vi "Destroy.vi"(8 "error in (no error)":errorcluster, 11 "RefTypedCircularBuffer in":refnum<class "RefTypedCircularBuffer.lvclass">) -> (0 "error out":errorcluster)   [LabVIEW 2024, in "RefTypedCircularBuffer.lvclass"]
uses:
  RefTypedCircularBuffer.lvclass
  RefTypedCircularBuffer.lvclass/RefTypedCircularBuffer.ctl
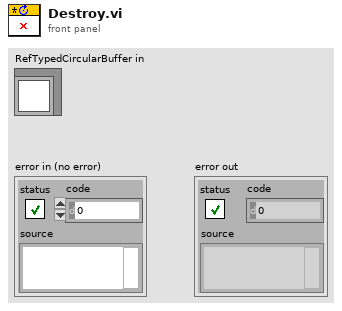
[diagram p1: front panel]
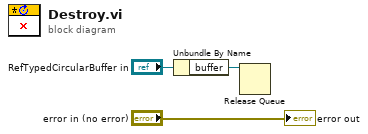
[diagram p0: block diagram]
diagram:
  n1 = Unbundle By Name("RefTypedCircularBuffer in") -> ("buffer"=w1:refnum<queue>)
  n2 = Release Queue(queue=w1) -> ()  [unwired: 2 in, 3 out]
  "error out" <- "error in (no error)"
